vi "Stop.vi"(8 "error in (no error)":errorcluster, 11 "Generate DC CFG in":refnum<class "Generate DC CFG.lvclass">) -> (0 "error out":errorcluster, 3 "Generate DC CFG out":refnum<class "Generate DC CFG.lvclass">)   [LabVIEW 2023, in "FGen Simulated CFGs.lvlib" / "Generate DC CFG.lvclass"]
uses:
  Generate DC CFG.lvclass
  Generate DC CFG.lvclass/Generate DC CFG.ctl
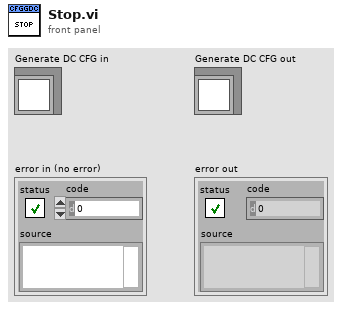
[diagram p1: front panel]
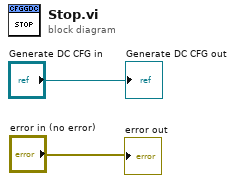
[diagram p0: block diagram]
diagram:
  "error out" <- "error in (no error)"
  "Generate DC CFG out" <- "Generate DC CFG in"
